vi "Shutdown.vi"(8 "error in":errorcluster, 11 "TCP master in":refnum<class "TCP Master.lvclass">) -> (0 "error out":errorcluster)   [LabVIEW 2021, in "TCP Master.lvclass"]
doc: "Closes the TCP connection stored in the class."
uses:
  TCP Master.lvclass
  D:/my_projects/projects/Algorithms/Labview/21/Modbus_v121c/Network Protocol/Network Master/Network Master.lvclass
  Network Master.lvclass/Network Master.ctl
  Transmission Data Unit/Transmission Data Unit.lvclass
  Network Master.lvclass
  TCP Master.lvclass/TCP Master.ctl
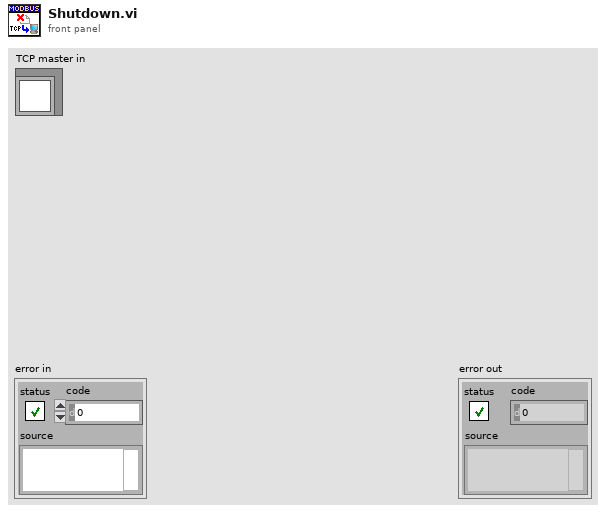
[diagram p1: front panel]
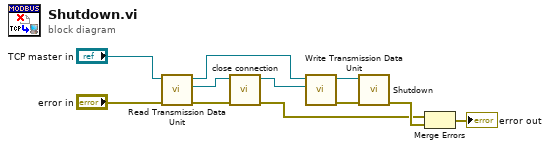
[diagram p0: block diagram]
diagram:
  n1 = call "Read Transmission Data Unit.vi"("error in (no error)"="error in", "Network Master in"="TCP master in") -> ("error out"=w6:errorcluster, "Transmission Data Unit"=w5:refnum<class "Transmission Data Unit.lvclass">, "Network Master out"=w9:refnum<class "TCP Master.lvclass">)  [unwired: 7 in]
  n2 = call-dynamic "close connection.vi"("error in"=w6, "transmission data unit in"=w5) -> ("error out"=w2:errorcluster, "transmission data unit out"=w4:refnum<class "Transmission Data Unit.lvclass">)  [unwired: 8 in]
  n3 = call "Write Transmission Data Unit.vi"("Transmission Data Unit"=w4, "Network Master in"=w9) -> ("error out"=w8:errorcluster, "Network Master out"=w7:refnum<class "TCP Master.lvclass">)  [unwired: 8 in]
  n4 = call-parent "Shutdown.vi"("error in"=w8, "Network Master in"=w7) -> ("error out"=w3:errorcluster)  [unwired: 9 in]
  n5 = Merge Errors(w2, w3) -> (→"error out":errorcluster)
